vi "Shutdown.vi"(8 "error in":errorcluster, 11 "Report Generator in":refnum<class "Report Generator.lvclass">) -> (0 "error out":errorcluster, 3 "Report Generator out":refnum<class "Report Generator.lvclass">)   [LabVIEW 2023, in "Report Generator.lvlib" / "Report Generator.lvclass"]
uses:
  Library/Report Generator.lvclass
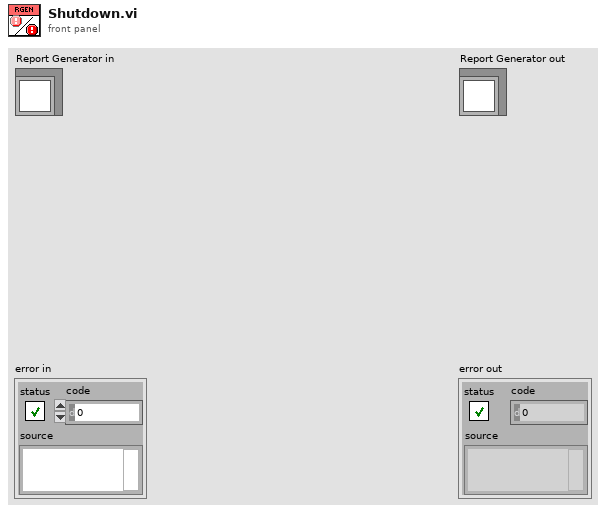
[diagram p1: front panel]
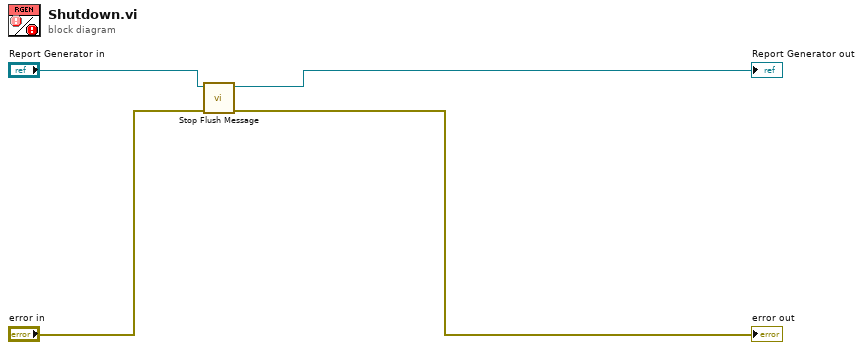
[diagram p0: block diagram]
diagram:
  n1 = call "Stop Flush Message.vi"("error in (no error)"="error in", "Report Generator in"="Report Generator in") -> ("error out"=→"error out":errorcluster, "Report Generator out"=→"Report Generator out":refnum<class "Report Generator.lvclass">)  [unwired: 8 in]
